vi "Autonomous Independent.vi"() -> ()   [LabVIEW 2014]
doc: "This VI is called when autonomous begins, and will automatically be terminated when autonomous ends. You can carry out timed or sensor driven robot movement independently without needing to return to the caller."
uses:
  <vilib>/Rock Robotics/WPI/Joystick/WPI_JoystickGetSetRefNum.vi
  <vilib>/Rock Robotics/WPI/RobotDrive/WPI_RobotDriveGetSetRefNum.vi
  <vilib>/Rock Robotics/WPI/RobotDrive/WPI_RobotDriveArcadeDrive_Standard(NoSaturation).vi
panel:
  out "Current Movement, for debugging":T1 {"Y Joystick Value" scale=1.0..-1.0; "X Joystick Value" scale=-1.0..1.0}
  in  "Array of robot movements":T2(array[cluster]) {"Y Joystick Value" scale=1.0..-1.0; "X Joystick Value" scale=-1.0..1.0}
  # "Be sure to right-click and choose Data Operations>>Make Current Value default if you want to save the array values with the VI"
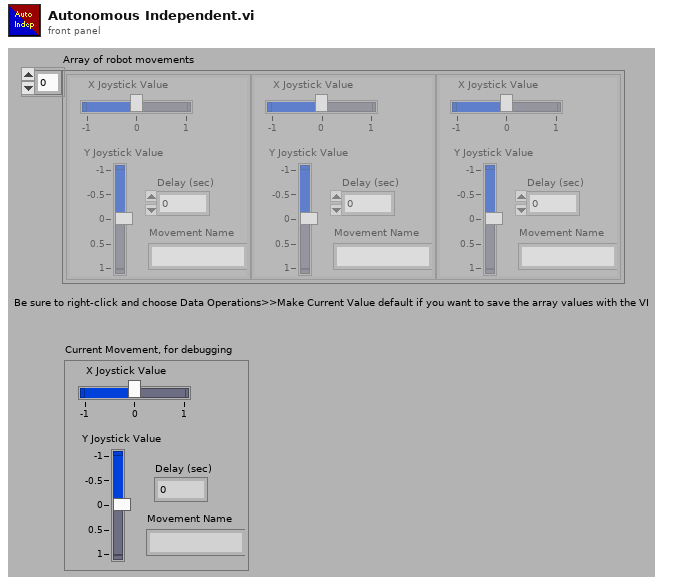
[diagram p1: front panel]
types:
  T1 = cluster{"X Joystick Value":dbl, "Y Joystick Value":dbl, "Delay (sec)":dbl, "Movement Name":string}
  T2 = cluster{"X Joystick Value":dbl, "Y Joystick Value":dbl, "Delay (sec)":dbl, "Movement Name":string}[]
  T3 = typedef "WPI_JoystickDevRef.ctl" = cluster{"Device":T4}
  T4 = typedef "WPI_JoystickDeviceEnum.ctl" = enum16{"USB 0", "USB 1", "USB 2", "USB 3", "USB 4", "USB 5"}
  T5 = typedef "WPI_RobotDriveDevRef.ctl" = cluster{"DevStatus":errorcluster, "Motors[]":T6[], "Square Inputs":bool, "Max Output":dbl}
  T6 = typedef "WPI_MotorControlDeviceRef.ctl" = cluster{"DeviceStatus":errorcluster, "Type":T7, "PWM":cluster{"Controller":T8, "PWM Channel":T9, "DeadBand":T10}, "CAN":cluster{"Device Number":u8, "Control Mode":T11, "Semaphore":T12, "Max Vout":dbl, "TalonSRX Control Mode":T13}, "Invert":bool, "TransformRef":T14, "InvTransformRef":T14}
  T7 = typedef "WPI_MotorControlType.ctl" = enum16{"PWM", "CAN", "CANTalonSRX"}
  T8 = typedef "FPGA_TypedefDigitalModule.ctl" = enum16{"Controller 1"}
  T9 = typedef "FPGA_DIOPWMChannel.ctl" = enum8{"PWM 0", "PWM 1", "PWM 2", "PWM 3", "PWM 4", "PWM 5", "PWM 6", "PWM 7", "PWM 8", "PWM 9", "PWM MXP 0", "PWM MXP 1", "PWM MXP 2", "PWM MXP 3", "PWM MXP 4", "PWM MXP 5", "PWM MXP 6", "PWM MXP 7", "PWM MXP 8", "PWM MXP 9", "Invalid"}
  T10 = typedef "WPI_PWMDeadband.ctl" = cluster{"Name":string, "maxPositivePwm":i32, "minPositivePwm":i32, "centerPwm":i32, "maxNegativePwm":i32, "minNegativePwm":i32, "angularRange":u16}
  T11 = typedef "WPI_CANJaguar_ControlMode.ctl" = enum8{"Percent VBus", "Current", "Speed", "Position", "Voltage"}
  T12 = typedef "Semaphore RefNum" = refnum<k1>
  T13 = typedef "WPI_CANTalonSRX_APIControlMode.ctl" = enum8{"Percent VBus", "Speed", "Position", "Slave", "Unchanged / Invalid"}
  T14 = typedef "WPI_PWMTransform_ConPane.ctl" = refnum<vi>
  T15 = typedef "WPI_EncoderDevRef.ctl" = cluster{"DevStatus":errorcluster, "EncoderIndex":T16, "CounterIndex":T17, "DistancePerCount":dbl, "Decoding Type":T18}
  T16 = typedef "FPGA_EncoderIdx.ctl" = enum8{"Enc 0", "Enc 1", "Enc 2", "Enc 3", "Enc 4", "Enc 5", "Enc 6", "Enc 7", "Invalid"}
  T17 = typedef "FPGA_CounterCtrSystemIndex.ctl" = enum8{"Ctr 0", "Ctr 1", "Ctr 2", "Ctr 3", "Ctr 4", "Ctr 5", "Ctr 6", "Ctr 7", "Invalid"}
  T18 = typedef "WPI_EncoderType.ctl" = enum16{"1x", "2x", "4x"}
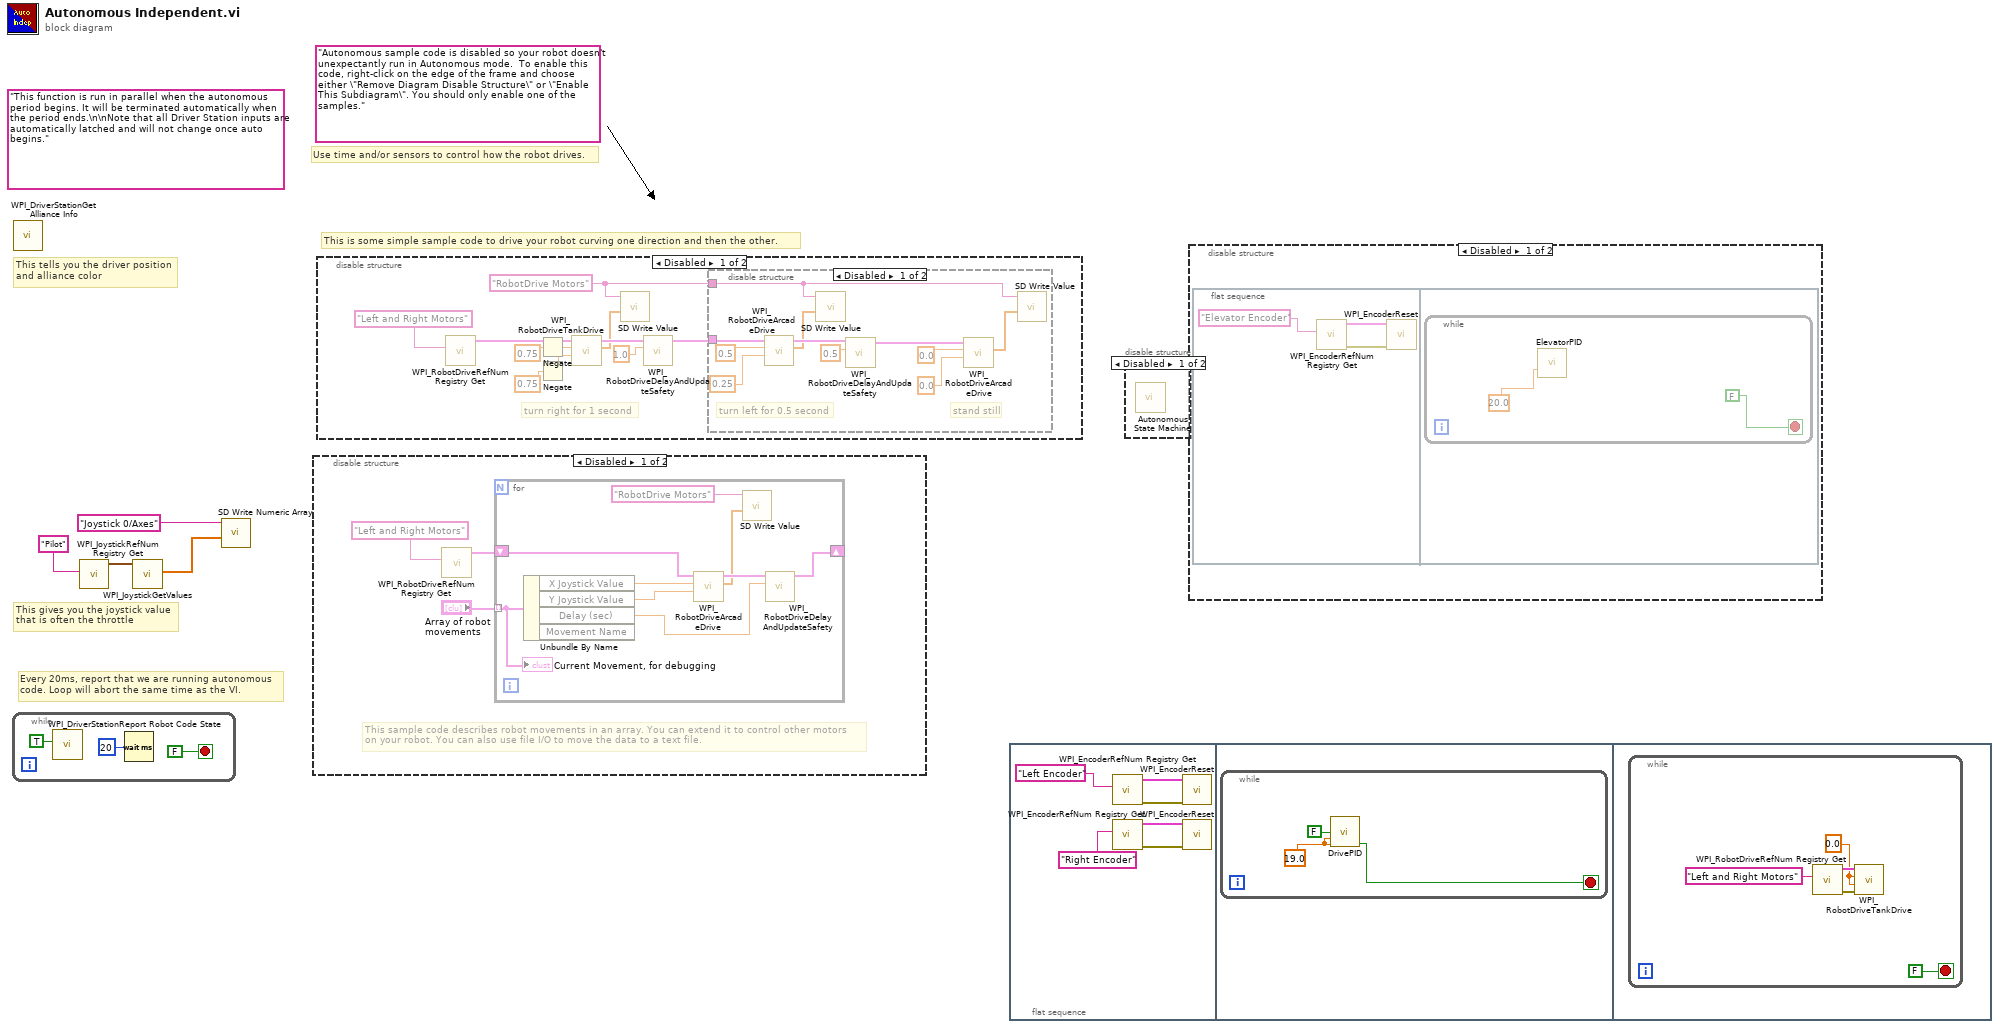
[diagram p0: block diagram]
diagram:
  (unwired) "Autonomous sample code is disabled so your robot doesn't unexpectantly run in Autonomous mode.  To enable this code, right-click on the edge of the frame and choose either \"Remove Diagram Disable Structure\" or \"Enable This Subdiagram\". You should only enable one of the samples."
  (unwired) "This function is run in parallel when the autonomous period begins. It will be terminated automatically when the period ends.\n\nNote that all Driver Station inputs are automatically latched and will not change once auto begins."
  # "This is some simple sample code to drive your robot curving one direction and then the other."
  # "Every 20ms, report that we are running autonomous\ncode. Loop will abort the same time as the VI."
  # "This gives you the joystick value\nthat is often the throttle"
  # "Use time and/or sensors to control how the robot drives."
  # "This tells you the driver position\nand alliance color"
  n1 = while {
    stop <- FALSE stop-if-true
    n2 = call <vilib>:"WPI_DriverStationReport Robot Code State.vi"("Autonomous"=TRUE) -> ()  [unwired: 10 in, 1 out]
    n3 = Wait (ms)(milliseconds to wait=u32 20) -> ()  [unwired: 1 out]
  }
  n4 = call <vilib>:"WPI_DriverStationGet Alliance Info.vi"() -> ()  [unwired: 12 out]
  n5 = call <vilib>:"WPI_JoystickRefNum Registry Get.vi"("refnum name"="Pilot") -> ("JoystickDevRef"=w3:T3)  [unwired: 1 in, 9 out]
  n6 = call <vilib>:"WPI_JoystickGetValues.vi"("JoystickDevRef"=w3) -> ("Axes"=w1:dbl[])  [unwired: 6 in, 4 out]
  n7 = call <vilib>:"SD Write Numeric Array.vi"("Numeric Array"=w1, "Name"="Joystick 0/Axes") -> ()  [unwired: 8 in, 2 out]
  n8 = disable-structure shown="Disabled" {
    frame Disabled {
      # "This sample code describes robot movements in an array. You can extend it to control other motors\non your robot. You can also use file I/O to move the data to a text file."
      n9 = call <vilib>:"WPI_RobotDriveRefNum Registry Get.vi"("refnum name"="Left and Right Motors") -> ("RobotDriveDevRef"=w9:T5)  [unwired: 1 in, 9 out]
      n10 = for {
        shift-right: [w16] -> _
        shift-left: w9 -> [w17]
        tunnel: "Array of robot movements" -> [w12] mode=indexing
        n11 = Unbundle By Name(w12) -> ("X Joystick Value"=w15:dbl, "Y Joystick Value"=w14:dbl, "Delay (sec)"=w13:dbl)  [unwired: 1 out]
        n12 = call-poly <vilib>:"WPI_RobotDriveArcadeDrive.vi"("Y axis value"=w14, "X axis value"=w15, "RobotDriveDevRef"=w17) -> ("Motor Values"=w11:dbl[], "RobotDriveDevRef"=w18:T5)  [unwired: 1 in, 6 out]
        n13 = call-poly <vilib>:"SD Write Value.vi"("Numeric Array"=w11, "Name"="RobotDrive Motors") -> ()  [unwired: 8 in, 2 out]
        n14 = call <vilib>:"WPI_RobotDriveDelayAndUpdateSafety.vi"("Delay (s)"=w13, "RobotDriveDevRef"=w18) -> ("RobotDriveDevRef 2"=w16:T5)  [unwired: 8 in, 1 out]
        "Current Movement, for debugging" <- w12
      }
    }
    frame Enabled {
    }
  }
  n15 = disable-structure shown="Disabled" {
    frame Disabled {
      w23 = "RobotDrive Motors" ("Name")
      # "turn right for 1 second"
      n16 = call <vilib>:"WPI_RobotDriveRefNum Registry Get.vi"("refnum name"="Left and Right Motors") -> ("RobotDriveDevRef"=w24:T5)  [unwired: 1 in, 9 out]
      n17 = Negate(x=0.75 ("X axis value")) -> (-x=w21:dbl)
      n18 = Negate(x=0.75 ("X axis value")) -> (-x=w20:dbl)
      n19 = call <vilib>:"WPI_RobotDriveTankDrive.vi"("Right axis value"=w20, "Left axis value"=w21, "RobotDriveDevRef"=w24) -> ("Motor Values"=w22:dbl[], "RobotDriveDevRef"=w28:T5)  [unwired: 6 in, 1 out]
      n20 = call-poly <vilib>:"SD Write Value.vi"("Numeric Array"=w22, "Name"=w23) -> ()  [unwired: 8 in, 2 out]
      n21 = call <vilib>:"WPI_RobotDriveDelayAndUpdateSafety.vi"("Delay (s)"=1.0, "RobotDriveDevRef"=w28) -> ("RobotDriveDevRef 2"=w27:T5)  [unwired: 8 in, 1 out]
      n22 = disable-structure shown="Disabled" {
        disable-tunnel: w27 -> [w37 _]
        disable-tunnel: w23 -> [w33 _]
        frame Disabled {
          # "stand still"
          # "turn left for 0.5 second"
          n23 = call-poly <vilib>:"WPI_RobotDriveArcadeDrive.vi"("Y axis value"=0.25 ("X axis value"), "X axis value"=0.5, "RobotDriveDevRef"=w37) -> ("Motor Values"=w32:dbl[], "RobotDriveDevRef"=w36:T5)  [unwired: 1 in, 6 out]
          n24 = call-poly <vilib>:"SD Write Value.vi"("Numeric Array"=w32, "Name"=w33) -> ()  [unwired: 8 in, 2 out]
          n25 = call <vilib>:"WPI_RobotDriveDelayAndUpdateSafety.vi"("Delay (s)"=0.5, "RobotDriveDevRef"=w36) -> ("RobotDriveDevRef 2"=w35:T5)  [unwired: 8 in, 1 out]
          n26 = call-poly <vilib>:"WPI_RobotDriveArcadeDrive.vi"("Y axis value"=0.0 ("X axis value"), "X axis value"=0.0, "RobotDriveDevRef"=w35) -> ("Motor Values"=w31:dbl[])  [unwired: 1 in, 7 out]
          n27 = call-poly <vilib>:"SD Write Value.vi"("Numeric Array"=w31, "Name"=w33) -> ()  [unwired: 8 in, 2 out]
        }
        frame Enabled {
        }
      }
    }
    frame Enabled {
    }
  }
  n28 = flat-sequence {
    frame #0 {
      n29 = call <vilib>:"WPI_EncoderRefNum Registry Get.vi"("refnum name"="Left Encoder") -> ("error out"=w47:errorcluster, "EncoderDevRef"=w46:T15)  [unwired: 9 in]
      n30 = call <vilib>:"WPI_EncoderRefNum Registry Get.vi"("refnum name"="Right Encoder") -> ("error out"=w45:errorcluster, "EncoderDevRef"=w44:T15)  [unwired: 9 in]
      n31 = call <vilib>:"WPI_EncoderReset.vi"("error in (no error)"=w47, "EncoderDevRef"=w46) -> ()  [unwired: 8 in, 2 out]
      n32 = call <vilib>:"WPI_EncoderReset.vi"("error in (no error)"=w45, "EncoderDevRef"=w44) -> ()  [unwired: 8 in, 2 out]
    }
    frame #1 {
      n33 = while {
        stop <- w48 stop-if-true
        w49 = 19.0 ("SetpointLeft")
        n34 = call "DrivePID.vi"("Compensate"=FALSE, "SetpointRight"=w49, "SetpointLeft"=w49) -> ("Done"=w48:bool)  [unwired: 12 in]
      }
    }
    frame #2 {
      n35 = while {
        stop <- FALSE stop-if-true
        w52 = 0.0 ("Left axis value")
        n36 = call <vilib>:"WPI_RobotDriveRefNum Registry Get.vi"("refnum name"="Left and Right Motors") -> ("error out"=w54:errorcluster, "RobotDriveDevRef"=w53:T5)  [unwired: 9 in]
        n37 = call <vilib>:"WPI_RobotDriveTankDrive.vi"("error in (no error)"=w54, "Right axis value"=w52, "Left axis value"=w52, "RobotDriveDevRef"=w53) -> ()  [unwired: 5 in, 3 out]
      }
    }
  }
  n38 = disable-structure shown="Disabled" {
    frame Disabled {
      n39 = call "Autonomous State Machine.vi"() -> ()  [unwired: 1 in]
    }
    frame Enabled {
    }
  }
  n40 = disable-structure shown="Disabled" {
    frame Disabled {
      n41 = flat-sequence {
        frame #0 {
          n42 = call <vilib>:"WPI_EncoderRefNum Registry Get.vi"("refnum name"="Elevator Encoder") -> ("error out"=w58:errorcluster, "EncoderDevRef"=w57:T15)  [unwired: 9 in]
          n43 = call <vilib>:"WPI_EncoderReset.vi"("error in (no error)"=w58, "EncoderDevRef"=w57) -> ()  [unwired: 8 in, 2 out]
        }
        frame #1 {
          n44 = while {
            stop <- FALSE stop-if-true
            n45 = call "ElevatorPID.vi"("Elevator Setpoint"=20.0 ("SetpointLeft")) -> ()  [unwired: 14 in, 1 out]
          }
        }
      }
    }
    frame Enabled {
    }
  }
